vi "pulse_width_modulation.vi"(5 "mAs":u32=950, 7 "Period (T)":dbl, 8 "error in (no error)":errorcluster, 9 "LED CHANNELS":dbl[](array[numeric]), 10 "LED_TABLE":dbl[][](array[numeric]), 11 "Iteration in":u32) -> (0 "ERROR OUT":errorcluster, 3 "Iteration out":u32)   [LabVIEW 2013]
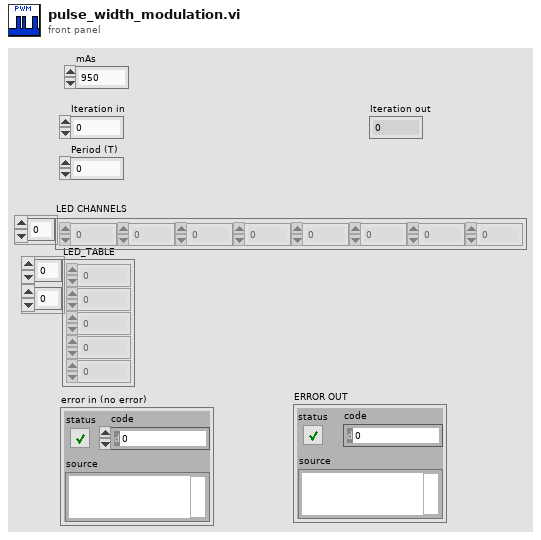
[diagram p1: front panel]
types:
  T1 = enum16{"Set Mode", "Set Normal Current ", "Set Strobe Parameters", "Set Normal Parameters", "Set Strobe Profile "}
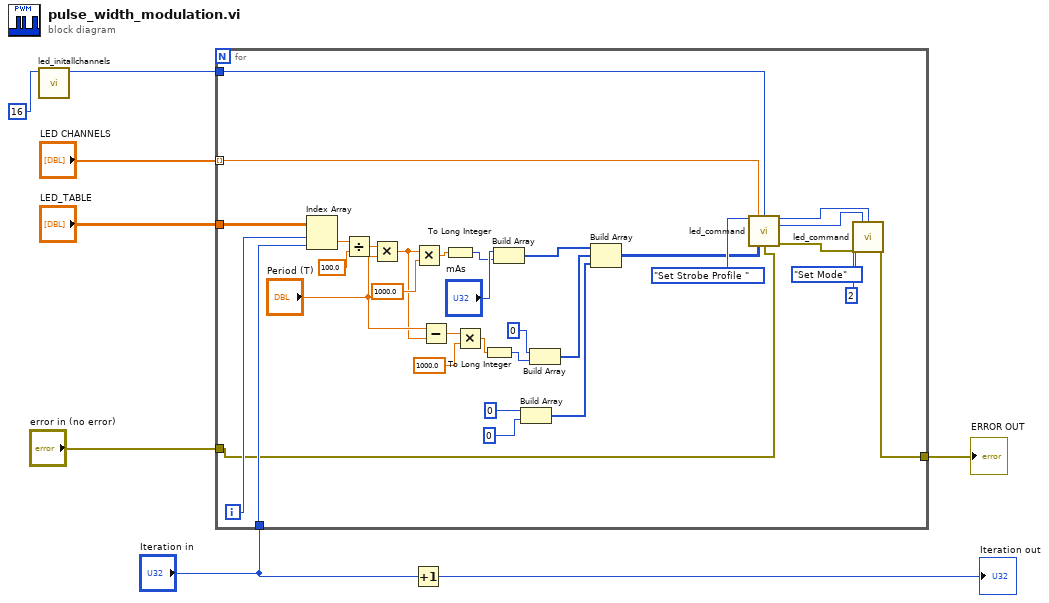
[diagram p0: block diagram]
diagram:
  n1 = call "led_initallchannels.vi"("Channels"=16) -> ("Device Handle Out"=w5:u32)  [unwired: 9 in, 1 out]
  n2 = for {
    tunnel: "LED_TABLE" -> [w41]
    tunnel: "Iteration in" -> [w39]
    tunnel: w5 -> [w38]
    tunnel: "LED CHANNELS" -> [w37] mode=indexing
    tunnel: "error in (no error)" -> [w29]
    tunnel: [w27] -> w2
    i -> [w40]
    n3 = Index Array(array=w41, index (row)=w40, index (col)=w39) -> (element=w21:dbl)
    n4 = Divide(x=w21, y=100.0) -> (x/y=w22:dbl)
    n5 = Multiply(x=w22, y="Period (T)") -> (x*y=w16:dbl)
    n6 = Multiply(x=w16, y=1000.0) -> (x*y=w18:dbl)
    n7 = Subtract(x="Period (T)", y=w16) -> (x-y=w14:dbl)
    n8 = To Long Integer(number=w18) -> (32bit integer=w11:i32)
    n9 = Multiply(x=w14, y=1000.0) -> (x*y=w15:dbl)
    n10 = To Long Integer(number=w15) -> (32bit integer=w10:i32)
    n11 = Build Array("mAs", w11) -> (w35:u32[])
    n12 = Build Array(0 ("element"), 0 ("element")) -> (w31:i32[])
    n13 = Build Array(0 ("element"), w10) -> (w34:i32[])
    n14 = Build Array(w35, w34, w31) -> (w30:u32[][])
    n15 = call "led_command.vi"("COMMAND"=T1."Set Strobe Profile ", "Channel"=w37, "Device Handle"=w38, "Strobe Profile"=w30, "ERROR"=w29) -> ("Device Handle Out"=w26:u32, "Channel Out"=w25:i32, "ERROR OUT"=w28:errorcluster)  [unwired: 7 in, 1 out]
    n16 = call "led_command.vi"("COMMAND"=T1."Set Mode", "Channel"=w25, "Device Handle"=w26, "Mode"=u32 2, "ERROR"=w28) -> ("ERROR OUT"=w27:errorcluster)  [unwired: 7 in, 3 out]
  }
  "ERROR OUT" <- w2
  n17 = Increment(x="Iteration in") -> (x+1=→"Iteration out":u32)
